vi "NATIONAL_INSTRUMENTS_TEMPLATE_model.vi"(9 "commandAction":T1, 10 "parameters":dbl[](array[numeric])=[1.0, 1.0, 3.0, 1.0, 1.0, 1.0, 4.0, 1.0], 11 "inputs":dbl[](array[numeric])=[0.0]) -> (2 "returnValue":i32, 3 "outputs":dbl[](array[numeric]))   [LabVIEW 2019]
uses:
  LV_ModelCallAction.ctl
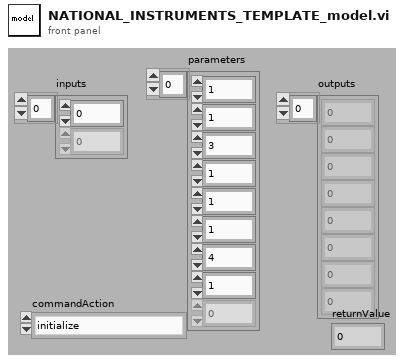
[diagram p1: front panel]
types:
  T1 = typedef "LV_ModelCallAction.ctl" = enum16{"initialize", "finalize", "normal"}
  T2 = enum16{"Runge-Kutta 1 (Euler)", "Runge-Kutta 2", "Runge-Kutta 3", "Runge-Kutta 4", "Runge-Kutta 23 (variable)", "Runge-Kutta 45 (variable)", "BDF (variable)", "Adams-Moulton (variable)", "Rosenbrock (variable)", "Discrete States Only"}
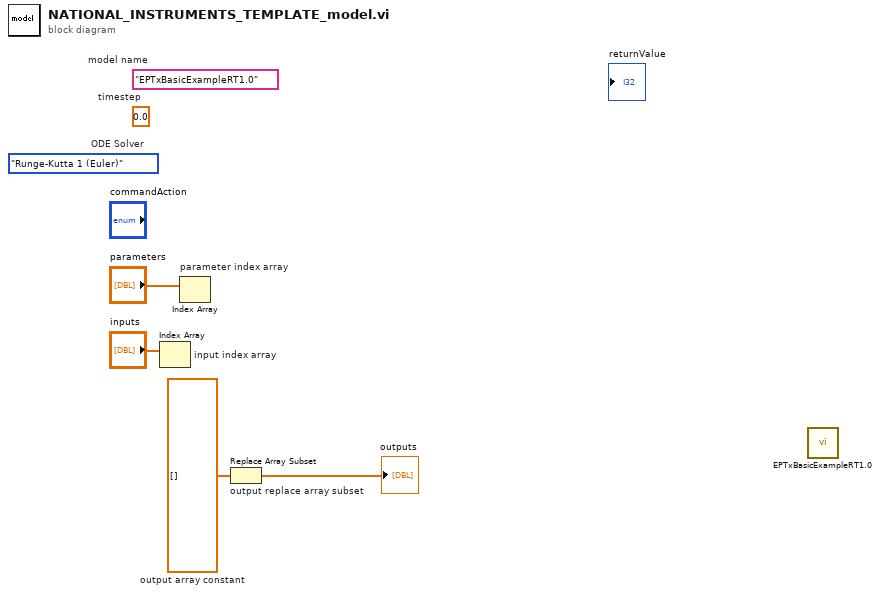
[diagram p0: block diagram]
diagram:
  (unwired) "EPTxBasicExampleRT1.0"  # model name
  (unwired) T2."Runge-Kutta 1 (Euler)"  # ODE Solver
  (unwired) 0.0  # timestep
  w2 = dbl[] []  # output array constant
  n1 = Index Array "input index array"(array="inputs") -> ()  [unwired: 1 in, 1 out]
  n2 = Index Array "parameter index array"(array="parameters") -> ()  [unwired: 1 in, 1 out]
  n3 = Replace Array Subset "output replace array subset"(array=w2) -> (→"outputs":dbl[])
  n4 = call "EPTxBasicExampleRT1.0.vi"() -> ()  [unwired: 12 in]
